vi "Read Is frontmost.vi"(9 "FPWindow in":refnum<class "FPWindow.lvclass">) -> (3 "FPWindow out":refnum<class "FPWindow.lvclass">, 4 "Is frontmost":bool)   [LabVIEW 2014, in "FPWindow.lvclass"]
uses:
  FPWindow.lvclass
  FPWindow.lvclass/FPWindow.ctl
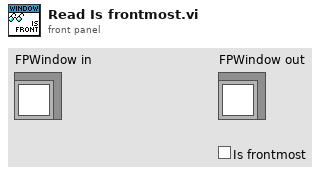
[diagram p1: front panel]
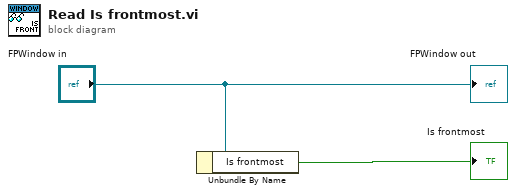
[diagram p0: block diagram]
diagram:
  n1 = Unbundle By Name("FPWindow in") -> ("Is frontmost"=→"Is frontmost":bool)
  "FPWindow out" <- "FPWindow in"
